vi "Create.vi"(8 "error in (no error)":errorcluster, 10 "VolatusAPI":refnum<class "VolatusAPI.lvclass">) -> (0 "error out":errorcluster, 3 "VolatusVariableResolver out":refnum<class "VolatusVariableResolver.lvclass">)   [LabVIEW 2020, in "Volatus.lvlib" / "VolatusVariableResolver.lvclass"]
uses:
  VolatusVariableResolver.lvclass
  VolatusVariableResolver.lvclass/VolatusVariableResolver.ctl
  VolatusAPI/VolatusAPI.lvclass
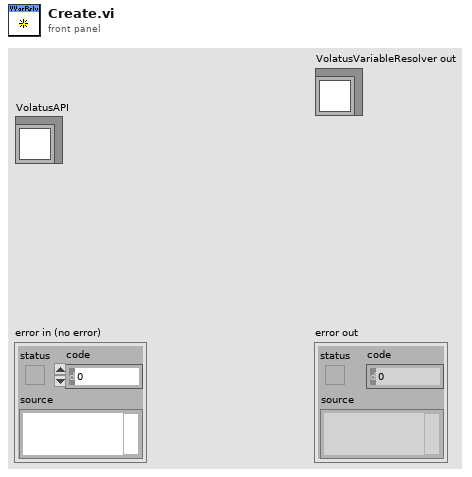
[diagram p1: front panel]
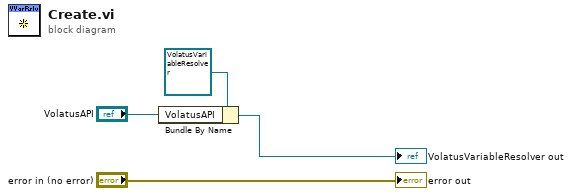
[diagram p0: block diagram]
diagram:
  n1 = Bundle By Name(cluster=refnum<class "VolatusVariableResolver.lvclass"> refnum ("VolatusVariableResolver in"), "VolatusAPI"="VolatusAPI") -> (→"VolatusVariableResolver out":refnum<class "VolatusVariableResolver.lvclass">)
  "error out" <- "error in (no error)"
